vi "DBGetFileList.vi"(5 "# of row (90)":i32=90, 7 "Days":i32, 8 "error in (no error)":errorcluster, 11 "ProcessState in":T2) -> (0 "error out":errorcluster, 1 "File For Delete":T1, 2 "Delete?":bool, 3 "ProcessState out":T2)   [LabVIEW 2015, in "FileHandler.lvlib"]
uses:
  FileHandler.lvlib
  controls/ProcessState.ctl
  <vilib>/drjdpowell/SQLite Library/SQL Connection/Connection.lvclass
  controls/FileForDelete.ctl
  <vilib>/Utility/miscctls.llb/LVDateTimeRec.ctl
  <vilib>/drjdpowell/SQLite Library/SQL Statement/SQL Statement.lvclass/SQL Statement.ctl
  <vilib>/drjdpowell/SQLite Library/SQL Statement/Bind Timestamp (Text).vi
  <vilib>/drjdpowell/SQLite Library/SQL Statement/Bind Text.vi
  <vilib>/drjdpowell/SQLite Library/SQL Statement/Error Message.vi
  <vilib>/drjdpowell/SQLite Library/SQL Statement/Column Timestamp.vi
  <vilib>/drjdpowell/SQLite Library/SQL Statement/Column String.vi
  <vilib>/drjdpowell/SQLite Library/SQL Statement/Column Path.vi
  DBToolkit/DBToolkit.lvlib
  <vilib>/drjdpowell/SQLite Library/SQL Statement/SQL Statement.lvclass
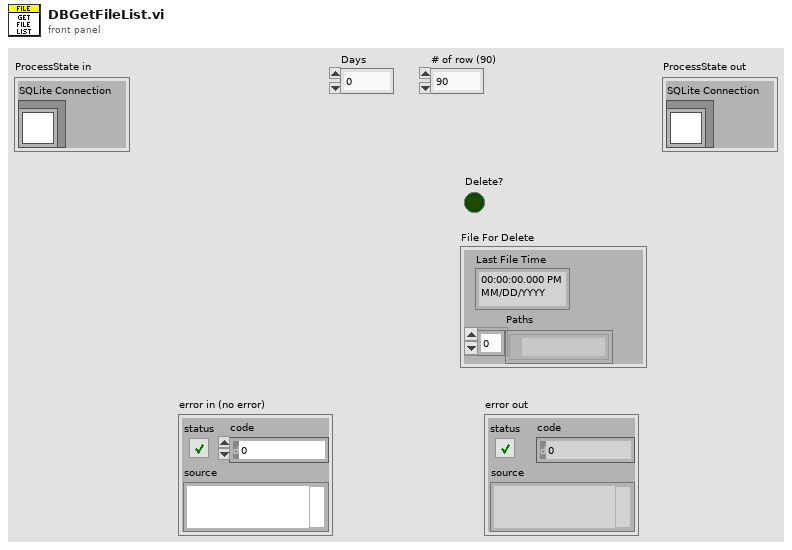
[diagram p1: front panel]
types:
  T1 = typedef "FileHandler.lvlib/FileForDelete.ctl" = cluster{"Last File Time":timestamp, "Paths":path[]}
  T2 = typedef "FileHandler.lvlib/ProcessState.ctl" = cluster{"SQLite Connection":refnum<class "Connection.lvclass">}
  T3 = typedef "LVDateTimeRec.ctl" = cluster{"fractional second":dbl, "second":i32, "minute":i32, "hour":i32, "day of month":i32, "month":i32, "year":i32, "day of week":i32, "day of year":i32, "DST":i32}
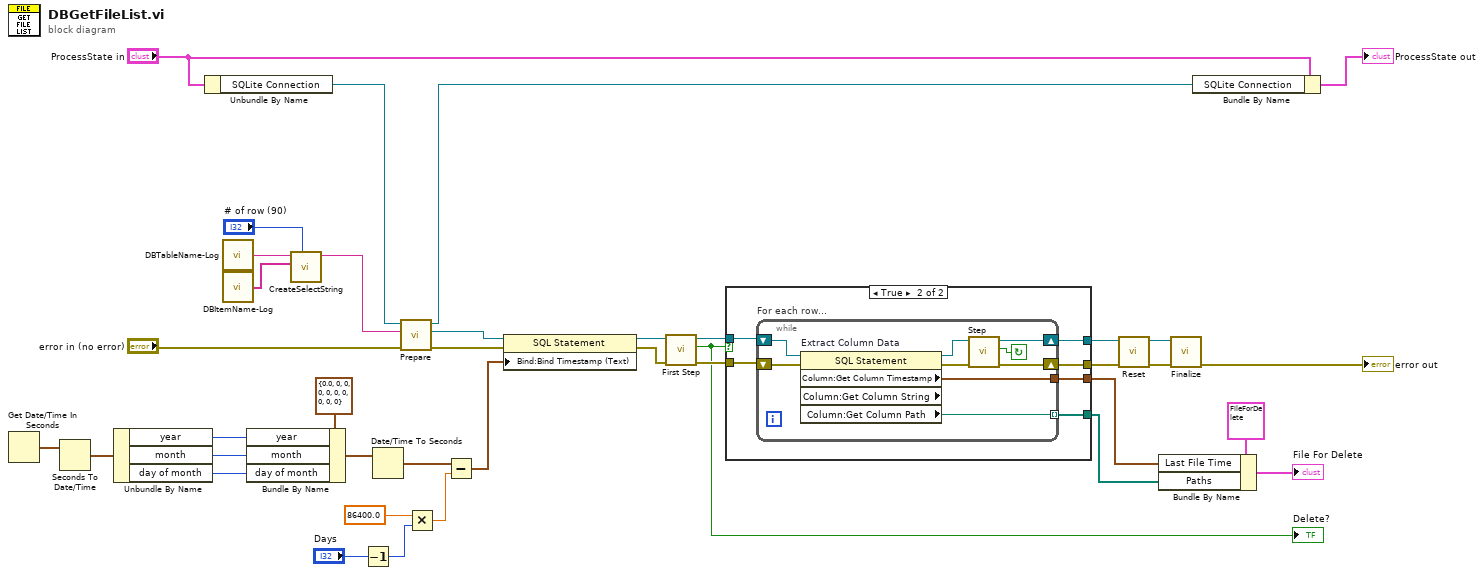
[diagram p0: block diagram]
diagram:
  n1 = Get Date/Time In Seconds() -> (seconds since 1Jan1904=w21:timestamp)
  n2 = Seconds To Date/Time(time stamp (now)=w21) -> (date time rec=w22:T3)  [unwired: 1 in]
  n3 = Unbundle By Name(w22) -> ("year"=w30:i32, "month"=w29:i32, "day of month"=w28:i32)
  n4 = Unbundle By Name("ProcessState in") -> ("SQLite Connection"=w34:refnum<class "Connection.lvclass">)
  n5 = call "DBTableName-Log.vi"() -> ("DB Table Name"=w33:string)  [unwired: 5 in]
  n6 = call "DBItemName-Log.vi"() -> ("Items"=w32:string[])  [unwired: 5 in]
  n7 = Bundle By Name(cluster=T3 {"fractional second"=0.0, "second"=0, "minute"=0, "hour"=0, "day of month"=0, "month"=0, "year"=0, "day of week"=0, "day of year"=0, "DST"=0} ("date time rec"), "year"=w30, "month"=w29, "day of month"=w28) -> (w27:T3)
  n8 = call "CreateSelectString.vi"("# of row (90)"="# of row (90)", "Items"=w32, "Table Name"=w33) -> ("Create Select String (by Time)"=w36:string)  [unwired: 8 in]
  n9 = Decrement(x="Days") -> (x-1=w1:i32)
  n10 = Date/Time To Seconds(2:w27) -> (0:w26:timestamp)  [unwired: 1 in]
  n11 = call <vilib>:"Prepare.vi"("error in (no error)"="error in (no error)", "SQL"=w36, "SQLite Connection in"=w34) -> ("error out"=w19:errorcluster, "SQL Statement out"=w20:refnum<class "SQL Statement.lvclass">, "SQLite Connection out"=w9:refnum<class "Connection.lvclass">)  [unwired: 4 in, 2 out]
  n12 = Multiply(x=86400.0, y=w1) -> (x*y=w23:dbl)
  n13 = Subtract(x=w26, y=w23) -> (x-y=w18:timestamp)
  n14 = property class="SQL Statement"(reference=w20, error in=w19, "Bind:Bind Timestamp (Text)"=w18) -> (reference out=w17:refnum<class "SQL Statement.lvclass">, error out=w16:errorcluster)
  n15 = call <vilib>:"First Step.vi"("error in (no error)"=w16, "SQL Statement in"=w17) -> ("error out"=w14:errorcluster, "Row returned"=w3:bool, "SQL Statement out"=w15:refnum<class "SQL Statement.lvclass">)  [unwired: 7 in]
  "Delete?" <- w3
  n16 = case shown="True" w3 {
    tunnel: w15 -> [w39 w46]
    tunnel: w14 -> [w40 w45]
    tunnel: [w40 w44] -> w10
    tunnel: [w39 w43] -> w11
    tunnel: [_ w42] -> w5
    tunnel: [_ w41] -> w6
    frame False {
    }
    frame True {
      n17 = while "For each row..." {
        shift-right: [w54] -> w43
        shift-left: w46 -> [w51]
        shift-right: [w52] -> w44
        shift-left: w45 -> [w50]
        tunnel: [w48] -> w41 mode=indexing
        tunnel: [w47] -> w42
        stop <- w49 continue-if-true
        n18 = property on="Extract Column Data" class="SQL Statement" props=["Column:Get Column Timestamp", "Column:Get Column String", "Column:Get Column Path"](reference=w51, error in=w50) -> (reference out=w55:refnum<class "SQL Statement.lvclass">, error out=w53:errorcluster, "Column:Get Column Timestamp"=w47:timestamp, "Column:Get Column Path"=w48:path)  [unwired: 1 out]
        n19 = call <vilib>:"Step.vi"("error in (no error)"=w53, "SQL Statement in"=w55) -> ("error out"=w52:errorcluster, "Row returned"=w49:bool, "SQL Statement out"=w54:refnum<class "SQL Statement.lvclass">)  [unwired: 7 in]
      }
    }
  }
  n20 = call <vilib>:"Reset.vi"("error in (no error)"=w10, "SQL Statement in"=w11) -> ("error out"=w12:errorcluster, "SQL Statement out"=w13:refnum<class "SQL Statement.lvclass">)  [unwired: 8 in]
  n21 = Bundle By Name(cluster=T1 {"Last File Time"=timestamp(0 s since 1904-01-01), "Paths"=[]} ("FileForDelete"), "Last File Time"=w5, "Paths"=w6) -> (→"File For Delete":T1)
  n22 = call <vilib>:"Finalize.vi"("error in (no error)"=w12, "SQL Statement in"=w13) -> ("error out"=→"error out":errorcluster)  [unwired: 9 in]
  n23 = Bundle By Name(cluster="ProcessState in", "SQLite Connection"=w9) -> (→"ProcessState out":T2)
